vi "_attribute_read_int32.vi"(5 "Repeated Capability":string, 7 "Attribute":T1={"Identifier"="", "Descriptive Name"="", "Data Type"=enum."Integer 32", "Command"="", "Access"=enum."Read/Write", "Range Table"="", "Read Callback"="", "Write Callback"="", "Supported Models"="", "Instrument Options"="", "Index"=0, "OPC Wait"=FALSE, "No Status Check"=FALSE, "Cache Only"=FALSE}, 8 "error in":errorcluster caption="error in (no error)", 10 "Query Parameter":string, 11 "VISA resource name":refnum<visa-resource-name>) -> (0 "error out":errorcluster, 2 "Int32 out":i32, 3 "VISA resource name out":refnum<visa-resource-name>)   [LabVIEW 2022 SP3, in "hmp4000_rsidr_core.lvlib"]
uses:
  hmp4000_rsidr_core.lvlib
  type_Attribute.ctl
  type_Attribute_Data_Type.ctl
  type_ReadWriteAccess.ctl
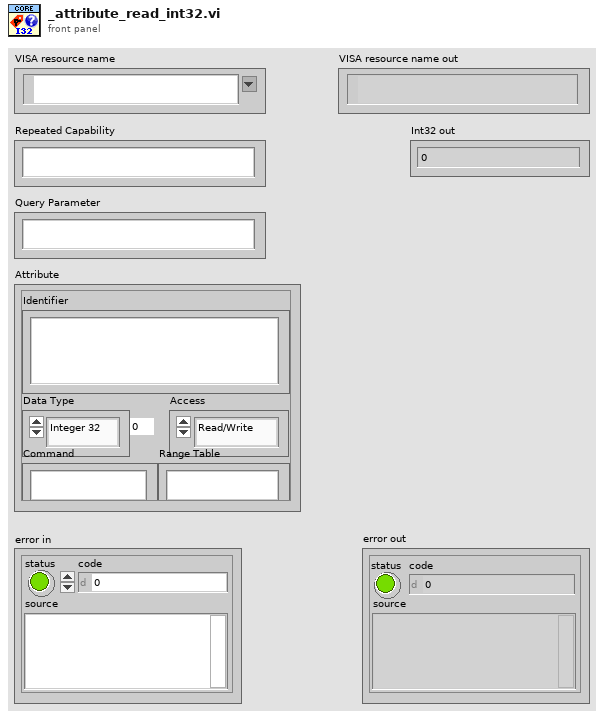
[diagram p1: front panel]
types:
  T1 = typedef "hmp4000_rsidr_core.lvlib/type_Attribute.ctl" = cluster{"Identifier":string, "Descriptive Name":string, "Data Type":T2, "Command":string, "Access":T3, "Range Table":string, "Read Callback":string, "Write Callback":string, "Supported Models":string, "Instrument Options":string, "Index":i32, "OPC Wait":bool, "No Status Check":bool, "Cache Only":bool}
  T2 = typedef "hmp4000_rsidr_core.lvlib/type_Attribute_Data_Type.ctl" = enum16{"Integer 32", "Double", "String", "Boolean", "None", "Integer 64", "RawString"}
  T3 = typedef "hmp4000_rsidr_core.lvlib/type_ReadWriteAccess.ctl" = enum16{"Read Only", "Write Only", "Read/Write"}
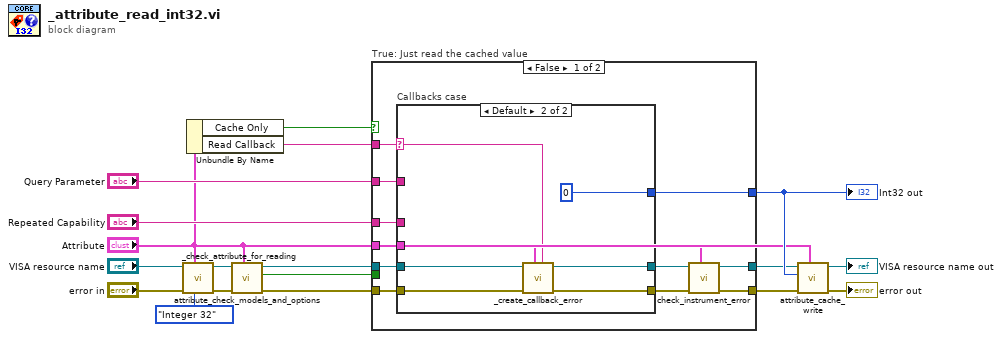
[diagram p0: block diagram]
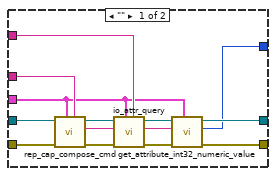
[diagram p2: hidden frame]
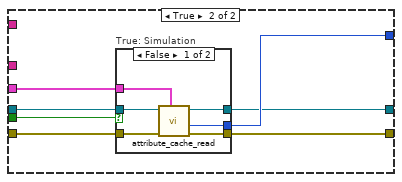
[diagram p3: hidden frame]
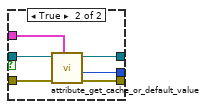
[diagram p4: hidden frame]
diagram:
  n1 = call "_check_attribute_for_reading.vi"("Expected Data Type"=type_Attribute_Data_Type."Integer 32" ("Data Type"), "Attribute"="Attribute", "error in"="error in", "VISA resource name"="VISA resource name") -> ("error out"=w9:errorcluster, "VISA resource name out"=w8:refnum<visa-resource-name>)  [unwired: 6 in]
  n2 = Unbundle By Name("Attribute") -> ("Cache Only"=w1:bool, "Read Callback"=w10:string)
  n3 = call "attribute_check_models_and_options.vi"("Attribute"="Attribute", "error in"=w9, "VISA resource name"=w8) -> ("error out"=w7:errorcluster, "Simulation Mode"=w5:bool, "VISA resource name out"=w6:refnum<visa-resource-name>)  [unwired: 6 in]
  n4 = case "True: Just read the cached value" shown="False" w1 {
    tunnel: "Repeated Capability" -> [w29 _]
    tunnel: [w21 w53] -> w4
    tunnel: [w20 w52] -> w3
    tunnel: [w28 w54] -> w13
    tunnel: w10 -> [w27 _]
    tunnel: w6 -> [w26 w56]
    tunnel: w7 -> [w25 w57]
    tunnel: "Attribute" -> [w19 w55]
    tunnel: "Query Parameter" -> [w24 _]
    tunnel: w5 -> [_ w51]
    frame False {
      n5 = case "Callbacks case" shown="Default" w27 {
        selector: w27 -> [_ w45]
        tunnel: w26 -> [w43 w49]
        tunnel: w25 -> [w42 w50]
        tunnel: w29 -> [w36 _]
        tunnel: [w41 w47] -> w22
        tunnel: [w40 w48] -> w23
        tunnel: [w33 0 ("Attribute Value I32")] -> w28
        tunnel: w19 -> [w30 w46]
        tunnel: w24 -> [w31 _]
        frame "" {
          n6 = call "rep_cap_compose_cmd.vi"("Repeated Capability"=w36, "Attribute"=w30, "error in"=w42, "VISA resource name"=w43) -> ("error out"=w39:errorcluster, "Command out"=w38:string, "VISA resource name out"=w37:refnum<visa-resource-name>)  [unwired: 5 in]
          n7 = call "io_attr_query.vi"("Query Parameter (None)"=w31, "Attribute"=w30, "error in"=w39, "write buffer"=w38, "VISA resource name"=w37) -> ("error out"=w35:errorcluster, "read buffer"=w32:string, "VISA resource name out"=w34:refnum<visa-resource-name>)  [unwired: 4 in]
          n8 = call "get_attribute_int32_numeric_value.vi"("Attribute"=w30, "error in"=w35, "Cmd Value in"=w32, "VISA resource name"=w34) -> ("error out"=w40:errorcluster, "Int32 value out"=w33:i32, "VISA resource name out"=w41:refnum<visa-resource-name>)  [unwired: 5 in]
        }
        frame Default {
          n9 = call "_create_callback_error.vi"("Callback Name"=w45, "Attribute"=w46, "error in"=w50, "VISA resource name"=w49) -> ("error out"=w48:errorcluster, "VISA resource name out"=w47:refnum<visa-resource-name>)  [unwired: 6 in]
        }
      }
      n10 = call "check_instrument_error.vi"("Attribute"=w19, "error in"=w23, "VISA resource name"=w22) -> ("error out"=w21:errorcluster, "VISA resource name out"=w20:refnum<visa-resource-name>)  [unwired: 7 in]
    }
    frame True {
      n11 = case "True: Simulation" shown="False" w51 {
        tunnel: w57 -> [w63 w69]
        tunnel: w56 -> [w62 w68]
        tunnel: w55 -> [w61 w64]
        tunnel: [w60 w65] -> w54
        tunnel: [w59 w67] -> w53
        tunnel: [w58 w66] -> w52
        frame False {
          n12 = call "attribute_cache_read.vi"("Attribute"=w61, "error in"=w63, "VISA resource name"=w62) -> ("error out"=w59:errorcluster, "Int32 out"=w60:i32, "VISA resource name out"=w58:refnum<visa-resource-name>)  [unwired: 1 in, 5 out]
        }
        frame True {
          n13 = call "attribute_get_cache_or_default_value.vi"("Attribute"=w64, "error in"=w69, "VISA resource name"=w68) -> ("error out"=w67:errorcluster, "Int32 out"=w65:i32, "VISA resource name out"=w66:refnum<visa-resource-name>)  [unwired: 1 in, 5 out]
        }
      }
    }
  }
  "Int32 out" <- w13
  n14 = call "attribute_cache_write.vi"("Attribute"="Attribute", "error in"=w4, "Value in"=w13, "VISA resource name"=w3) -> ("error out"=→"error out":errorcluster, "VISA resource name out"=→"VISA resource name out":refnum<visa-resource-name>)  [unwired: 6 in]
